vi "ErrorHandling.Fglb.vi"(7 "Action":T3=enum."get", 8 "error in (no error)":errorcluster, 10 "Error in":T1, 11 "Event source":T2) -> (0 "error out":errorcluster, 1 "changed":bool, 2 "Errors out":T1[](array[typedef]))   [LabVIEW 2016]
uses:
  ErrorHandling.Fglb.Action.ctl
  EventLog/EventLog.EventSource.ctl
  CitTemplate/citTemplate.errData.ctl
panel:
  out "Errors":T1[](array[typedef])
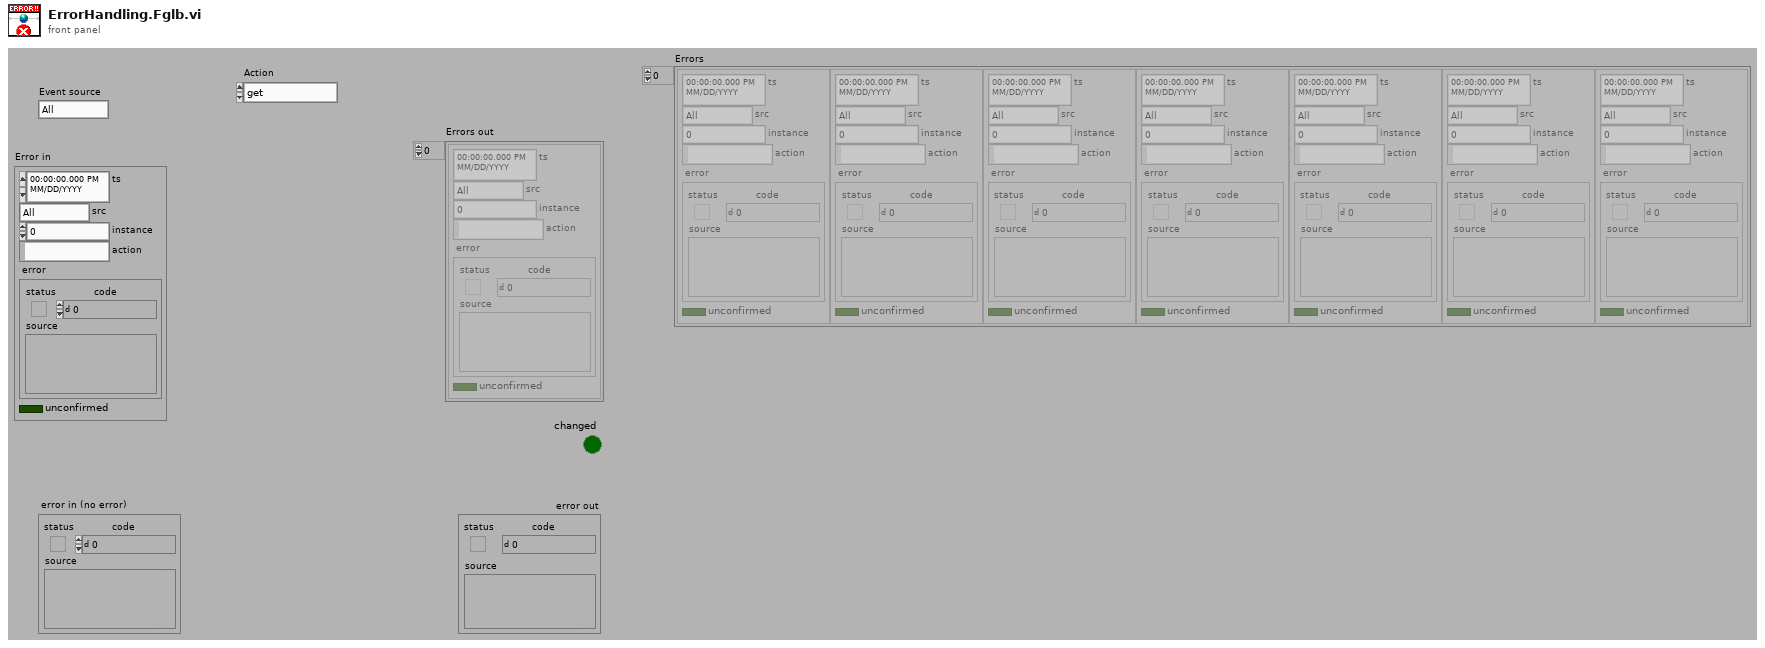
[diagram p1: front panel]
types:
  T1 = typedef "citTemplate.errData.ctl" = cluster{"ts":timestamp, "src":T2, "instance":i32, "action":string, "error":errorcluster, "unconfirmed":bool}
  T2 = typedef "EventLog.EventSource.ctl" = enum16{"All", "Gui", "Cache", "PLC1", "PLC2", "PLC3", "DB", "DB01", "DB02", "DB03", "DB04", "DB05", "DB06", "DB07", "DB08", "DB09", "DB10", "DB11", "DB12", "DB13", "DB14", "DB15", "DB16"}
  T3 = typedef "ErrorHandling.Fglb.Action.ctl" = enum16{"init", "add", "clear", "confirm", "check", "get"}
  T4 = cluster{"src":T2, "instance":i32, "action":string, "code":i32}
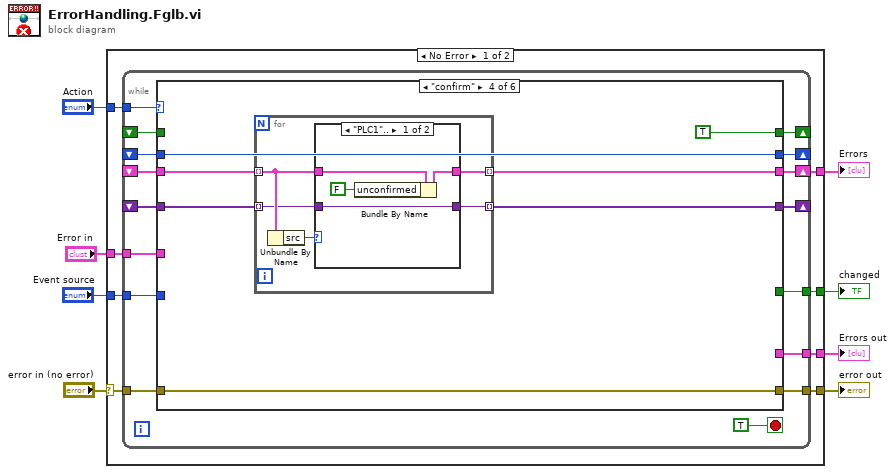
[diagram p0: block diagram]
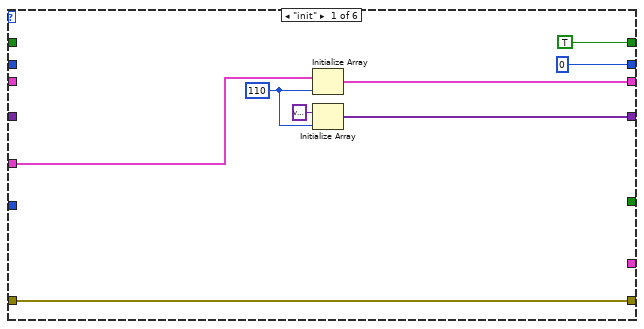
[diagram p2: hidden frame]
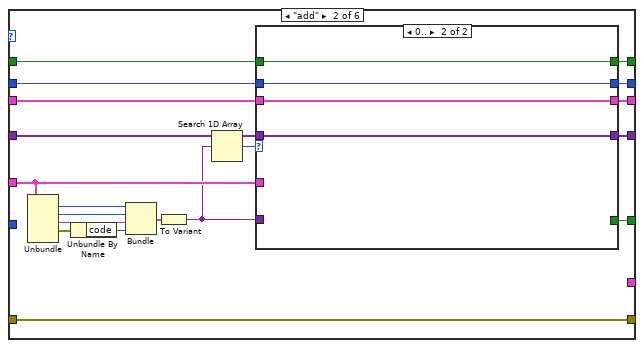
[diagram p3: hidden frame]
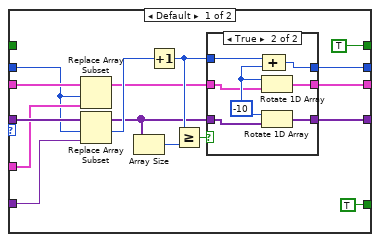
[diagram p4: hidden frame]
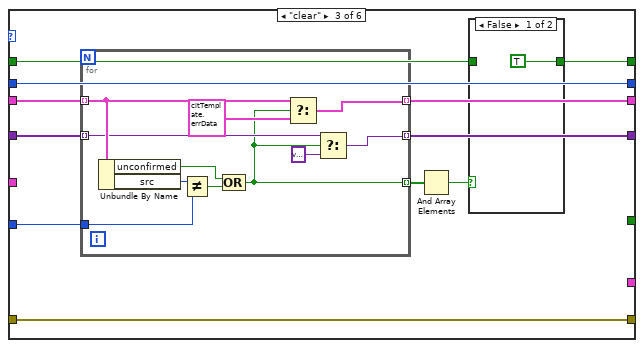
[diagram p6: hidden frame]
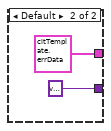
[diagram p8: hidden frame]
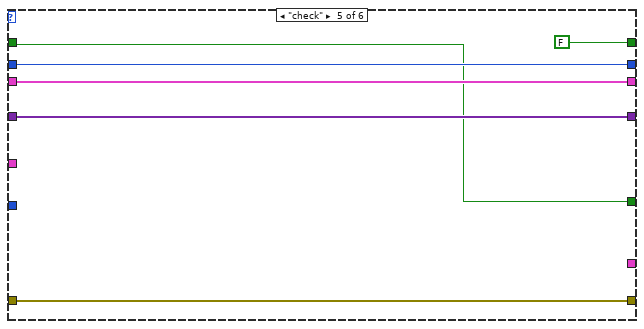
[diagram p9: hidden frame]
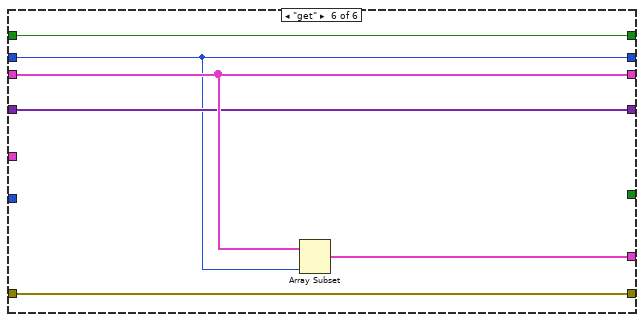
[diagram p10: hidden frame]
diagram:
  n1 = case shown="No Error" "error in (no error)" {
    selector: "error in (no error)" -> [w16 w143]
    tunnel: [w13 w143] -> w7
    tunnel: "Action" -> [w15 _]
    tunnel: "Error in" -> [w14 _]
    tunnel: "Event source" -> [w12 _]
    tunnel: [w11 _] -> w4
    tunnel: [w10 _] -> w3
    tunnel: [w9 _] -> w1
    frame No Error {
      n2 = while {
        tunnel: w16 -> [w27]
        tunnel: w15 -> [w32]
        tunnel: w14 -> [w31]
        shift-right: [w30] -> w10
        shift-left: _ -> [w29]
        tunnel: [w26] -> w13
        tunnel: w12 -> [w25]
        shift-right: [w24] -> _
        shift-left: _ -> [w23]
        tunnel: [w22] -> w11
        shift-right: [w21] -> _
        shift-left: _ -> [w20]
        shift-right: [w19] -> _
        shift-left: _ -> [w18]
        tunnel: [w17] -> w9
        stop <- TRUE stop-if-true
        n3 = case shown="\"confirm\"" w32 {
          tunnel: w31 -> [w40 w46 _ _ _ _]
          tunnel: [w38 w59 w99 w119 w133 w140] -> w30
          tunnel: w29 -> [_ w57 w98 w118 w133 w140]
          tunnel: w27 -> [w39 w58 w97 w117 w136 w142]
          tunnel: [w39 w58 w97 w117 w136 w142] -> w26
          tunnel: w25 -> [_ _ w96 _ _ _]
          tunnel: [TRUE w56 w89 TRUE FALSE w141] -> w24
          tunnel: w23 -> [_ w55 w92 _ w131 w141]
          tunnel: [_ _ _ _ _ w139] -> w22
          tunnel: [w34 w44 w93 w114 w134 w138] -> w21
          tunnel: w20 -> [_ w45 w94 w115 w134 w138]
          tunnel: [0 w48 w95 w113 w132 w137] -> w19
          tunnel: w18 -> [_ w49 w95 w113 w132 w137]
          tunnel: [_ w42 _ _ w131 _] -> w17
          frame "init" {
            w36 = 110 ("dimension size")
            n4 = Initialize Array(w40, w36) -> (w38:T1[])
            n5 = Initialize Array(variant ("variant"), w36) -> (w34:variant[])
          }
          frame "add" {
            n6 = Unbundle(w46) -> ("src"=w54:T2, "instance"=w53:i32, "action"=w52:string, "error"=w51:errorcluster)  [unwired: 2 out]
            n7 = Unbundle By Name(w51) -> ("code"=w41:i32)
            n8 = Bundle("src"=w54, "instance"=w53, "action"=w52, "code"=w41) -> (w50:T4)  [unwired: 1 in]
            n9 = To Variant(anything=w50) -> (Variant=w43:variant)
            n10 = Search 1D Array(1D array=w45, element=w43) -> (index of element=w47:i32)  [unwired: 1 in]
            n11 = case shown="0.." w47 {
              tunnel: [w62 w88] -> w59
              tunnel: w57 -> [w71 w88]
              tunnel: [TRUE w87] -> w56
              tunnel: w55 -> [_ w87]
              tunnel: w49 -> [w66 w86]
              tunnel: [w61 w86] -> w48
              tunnel: w46 -> [w72 _]
              tunnel: w45 -> [w73 w85]
              tunnel: [w64 w85] -> w44
              tunnel: w43 -> [w67 _]
              tunnel: [TRUE _] -> w42
              frame Default {
                n12 = Replace Array Subset(array=w71, new element=w72, index=w66) -> (w63:T1[])
                n13 = Replace Array Subset(array=w73, new element=w67, index=w66) -> (w65:variant[])
                n14 = Array Size(array=w65) -> (size(s)=w70:i32)
                n15 = Increment(x=w66) -> (x+1=w68:i32)
                n16 = Greater Or Equal?(x=w68, y=w70) -> (x >= y?=w69:bool)
                n17 = case shown="True" w69 {
                  tunnel: w68 -> [w76 w84]
                  tunnel: w65 -> [w75 w78]
                  tunnel: [w75 w83] -> w64
                  tunnel: [w76 w82] -> w61
                  tunnel: w63 -> [w77 w79]
                  tunnel: [w77 w81] -> w62
                  frame False {
                  }
                  frame True {
                    w80 = -10 ("y")
                    n18 = Rotate 1D Array(1:w79, 2:w80) -> (0:w81:T1[])
                    n19 = Rotate 1D Array(1:w78, 2:w80) -> (0:w83:variant[])
                    n20 = Compound Arithmetic op=ADD(w84, w80) -> (w82:i32)
                  }
                }
              }
              frame 0.. {
              }
            }
          }
          frame "clear" {
            n21 = for {
              tunnel: [w108] -> w99 mode=indexing
              tunnel: w98 -> [w109] mode=indexing
              tunnel: w96 -> [w112]
              tunnel: w94 -> [w107] mode=indexing
              tunnel: [w105] -> w93 mode=indexing
              tunnel: [w102] -> w91 mode=indexing
              n22 = Unbundle By Name(w109) -> ("unconfirmed"=w103:bool, "src"=w111:T2)
              n23 = Not Equal?(x=w111, y=w112) -> (x != y?=w106:bool)
              n24 = Compound Arithmetic op=OR(w103, w106) -> (w102:bool)
              n25 = Select(t=w109, s=w102, f=T1 {"ts"=timestamp(0 s since 1904-01-01), "src"=enum."All", "instance"=0, "action"="", "error"={"status"=FALSE, "code"=0, "source"=""}, "unconfirmed"=FALSE} ("new element/subarray")) -> (s? t:f=w108:T1)
              n26 = Select(t=w107, s=w102, f=variant) -> (s? t:f=w105:variant)
            }
            n27 = And Array Elements(Boolean array=w91) -> (logical AND=w90:bool)
            n28 = case shown="False" w90 {
              tunnel: w92 -> [_ w101]
              tunnel: [TRUE w101] -> w89
              frame False {
              }
              frame True {
              }
            }
          }
          frame "confirm" {
            n29 = for {
              tunnel: [w124] -> w119 mode=indexing
              tunnel: w118 -> [w123] mode=indexing
              tunnel: w115 -> [w121] mode=indexing
              tunnel: [w120] -> w114 mode=indexing
              n30 = Unbundle By Name(w123) -> ("src"=w122:T2)
              n31 = case shown="\"PLC1\".." w122 {
                tunnel: [w127 T1 {"ts"=timestamp(0 s since 1904-01-01), "src"=enum."All", "instance"=0, "action"="", "error"={"status"=FALSE, "code"=0, "source"=""}, "unconfirmed"=FALSE} ("new element/subarray")] -> w124
                tunnel: w123 -> [w128 _]
                tunnel: w121 -> [w125 _]
                tunnel: [w125 variant ("f")] -> w120
                frame "PLC1".. {
                  n32 = Bundle By Name(cluster=w128, "unconfirmed"=FALSE) -> (w127:T1)
                }
                frame Default {
                }
              }
            }
          }
          frame "check" {
          }
          frame "get" {
            n33 = Array Subset(array=w140, length=w137) -> (w139:T1[])  [unwired: 1 in]
          }
        }
      }
    }
    frame Error {
    }
  }
  "error out" <- w7
  "Errors out" <- w4
  "Errors" <- w3
  "changed" <- w1
